vi "create_test_log_folder.vi"(8 "error in (no error)":errorcluster, 10 "names in":T2) -> (0 "error out":errorcluster, 2 "fldr paths":T1)   [LabVIEW 2015]
doc: "This vi creates (if they do not exist) the test log folder (C:\\LogFiles), the accepted files folder (C:\\LogFiles\\accepted) and the rejected files folder (C:\\LogFiles\\rejected)"
uses:
  Type Definitions/created_folders_path.ctl
  <vilib>/Utility/error.llb/Error Cluster From Error Code.vi
  <vilib>/ErrorRing/Error Ring.xnode
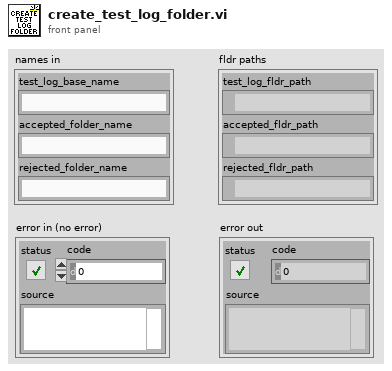
[diagram p1: front panel]
types:
  T1 = typedef "created_folders_path.ctl" = cluster{"test_log_fldr_path":path, "accepted_fldr_path":path, "rejected_fldr_path":path}
  T2 = cluster{"test_log_base_name":string, "accepted_folder_name":string, "rejected_folder_name":string}
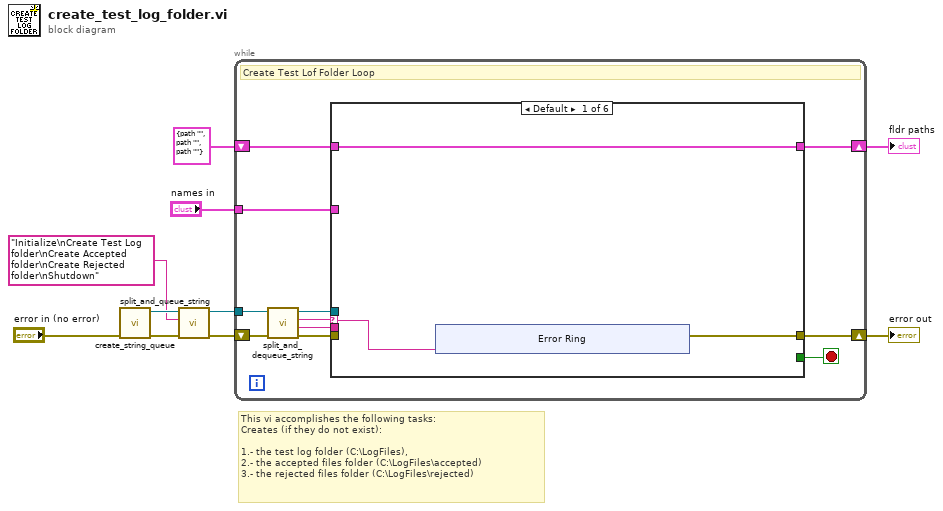
[diagram p0: block diagram]
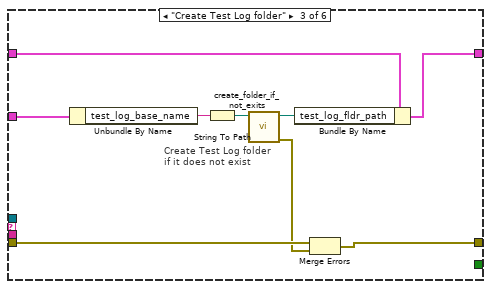
[diagram p3: hidden frame]
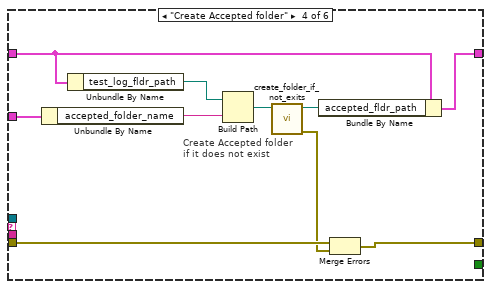
[diagram p4: hidden frame]
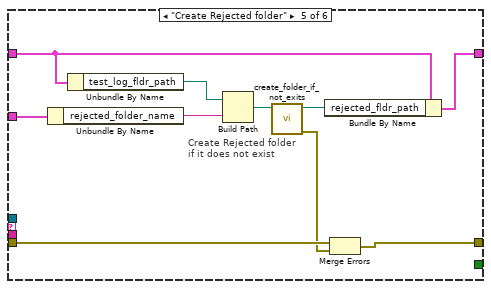
[diagram p5: hidden frame]
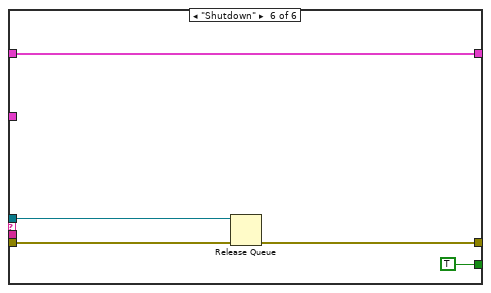
[diagram p6: hidden frame]
diagram:
  # "This vi accomplishes the following tasks:\nCreates (if they do not exist): \n\n1.- the test log folder (C:\\LogFiles), \n2.- the accepted files folder (C:\\LogFiles\\accepted)\n3.- the rejected files folder (C:\\LogFiles\\rejected)"
  n1 = call "create_string_queue.vi"("error in (no error)"="error in (no error)") -> ("error out"=w3:errorcluster, "Queue out"=w2:refnum<queue>)  [unwired: 9 in]
  n2 = call "split_and_queue_string.vi"("error in (no error)"=w3, "list state:argument"="Initialize\nCreate Test Log folder\nCreate Accepted folder\nCreate Rejected folder\nShutdown", "Queue in"=w2) -> ("error out"=w6:errorcluster, "Queue out"=w7:refnum<queue>)  [unwired: 7 in]
  n3 = while {
    shift-right: [w21] -> w9
    shift-left: w6 -> [w15]
    tunnel: "names in" -> [w19]
    tunnel: w7 -> [w16]
    shift-right: [w18] -> w8
    shift-left: T1 {"test_log_fldr_path"=path "", "accepted_fldr_path"=path "", "rejected_fldr_path"=path ""} ("paths out 2") -> [w17]
    stop <- w20 stop-if-true
    # "Create Test Lof Folder Loop"
    n4 = call "split_and_dequeue_string.vi"("error in (no error)"=w15, "Queue in"=w16) -> ("error out"=w11:errorcluster, "argument"=w12:string, "state"=w13:string, "Queue out"=w14:refnum<queue>)  [unwired: 6 in]
    n5 = case shown="Default" w13 {
      selector: w13 -> [w23 _ _ _ _ _]
      tunnel: w11 -> [_ w33 w40 w50 w59 w64]
      tunnel: [w22 w33 w39 w49 w58 w63] -> w21
      tunnel: [_ _ _ _ _ TRUE] -> w20
      tunnel: w19 -> [_ _ w41 w51 w60 _]
      tunnel: [w24 w32 w34 w46 w56 w66] -> w18
      tunnel: w14 -> [_ _ _ _ _ w65]
      tunnel: w17 -> [w24 w32 w35 w44 w54 w66]
      tunnel: w12 -> [_ _ _ _ _ _]
      frame Default {
        n6 = xnode "Error Ring"("parameter 0"=w23) -> ("error out"=w22:errorcluster)
      }
      frame "Initialize" {
      }
      frame "Create Test Log folder" {
        # "Create Test Log folder\nif it does not exist"
        n7 = Unbundle By Name(w41) -> ("test_log_base_name"=w42:string)
        n8 = String To Path(string=w42) -> (path=w38:path)
        n9 = call "create_folder_if_not_exits.vi"("appended path"=w38) -> ("error out"=w37:errorcluster, "created folder path"=w36:path)  [unwired: 9 in]
        n10 = Bundle By Name(cluster=w35, "test_log_fldr_path"=w36) -> (w34:T1)
        n11 = Merge Errors(w40, w37) -> (w39:errorcluster)
      }
      frame "Create Accepted folder" {
        # "Create Accepted folder\nif it does not exist"
        n12 = Unbundle By Name(w51) -> ("accepted_folder_name"=w52:string)
        n13 = Unbundle By Name(w44) -> ("test_log_fldr_path"=w43:path)
        n14 = Build Path(base path=w43, name or relative path=w52) -> (appended path=w48:path)
        n15 = call "create_folder_if_not_exits.vi"("appended path"=w48) -> ("error out"=w47:errorcluster, "created folder path"=w45:path)  [unwired: 9 in]
        n16 = Bundle By Name(cluster=w44, "accepted_fldr_path"=w45) -> (w46:T1)
        n17 = Merge Errors(w50, w47) -> (w49:errorcluster)
      }
      frame "Create Rejected folder" {
        # "Create Rejected folder\nif it does not exist"
        n18 = Unbundle By Name(w60) -> ("rejected_folder_name"=w62:string)
        n19 = Unbundle By Name(w54) -> ("test_log_fldr_path"=w53:path)
        n20 = Build Path(base path=w53, name or relative path=w62) -> (appended path=w61:path)
        n21 = call "create_folder_if_not_exits.vi"("appended path"=w61) -> ("error out"=w57:errorcluster, "created folder path"=w55:path)  [unwired: 9 in]
        n22 = Bundle By Name(cluster=w54, "rejected_fldr_path"=w55) -> (w56:T1)
        n23 = Merge Errors(w59, w57) -> (w58:errorcluster)
      }
      frame "Shutdown" {
        n24 = Release Queue(queue=w65, error in (no error)=w64) -> (error out=w63:errorcluster)  [unwired: 1 in, 2 out]
      }
    }
  }
  "error out" <- w9
  "fldr paths" <- w8
